vi "数字量输出自动检测_fast.vi"(11 "测试值":enum16{"0", "1"}(ring)) -> ()   [LabVIEW 2010]
uses:
  全局量/试验配置信息.vi
panel:
  in  "CAN端口":u16
  out "结束？":bool
  in  "同步_2":i32
  in  "同步_1":i32
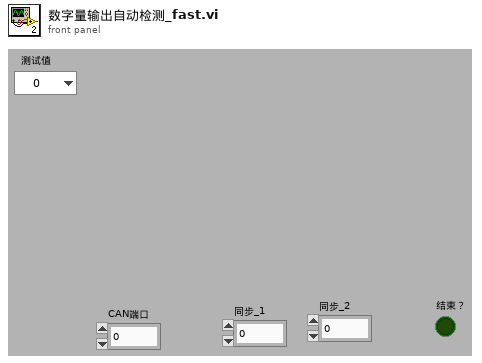
[diagram p1: front panel]
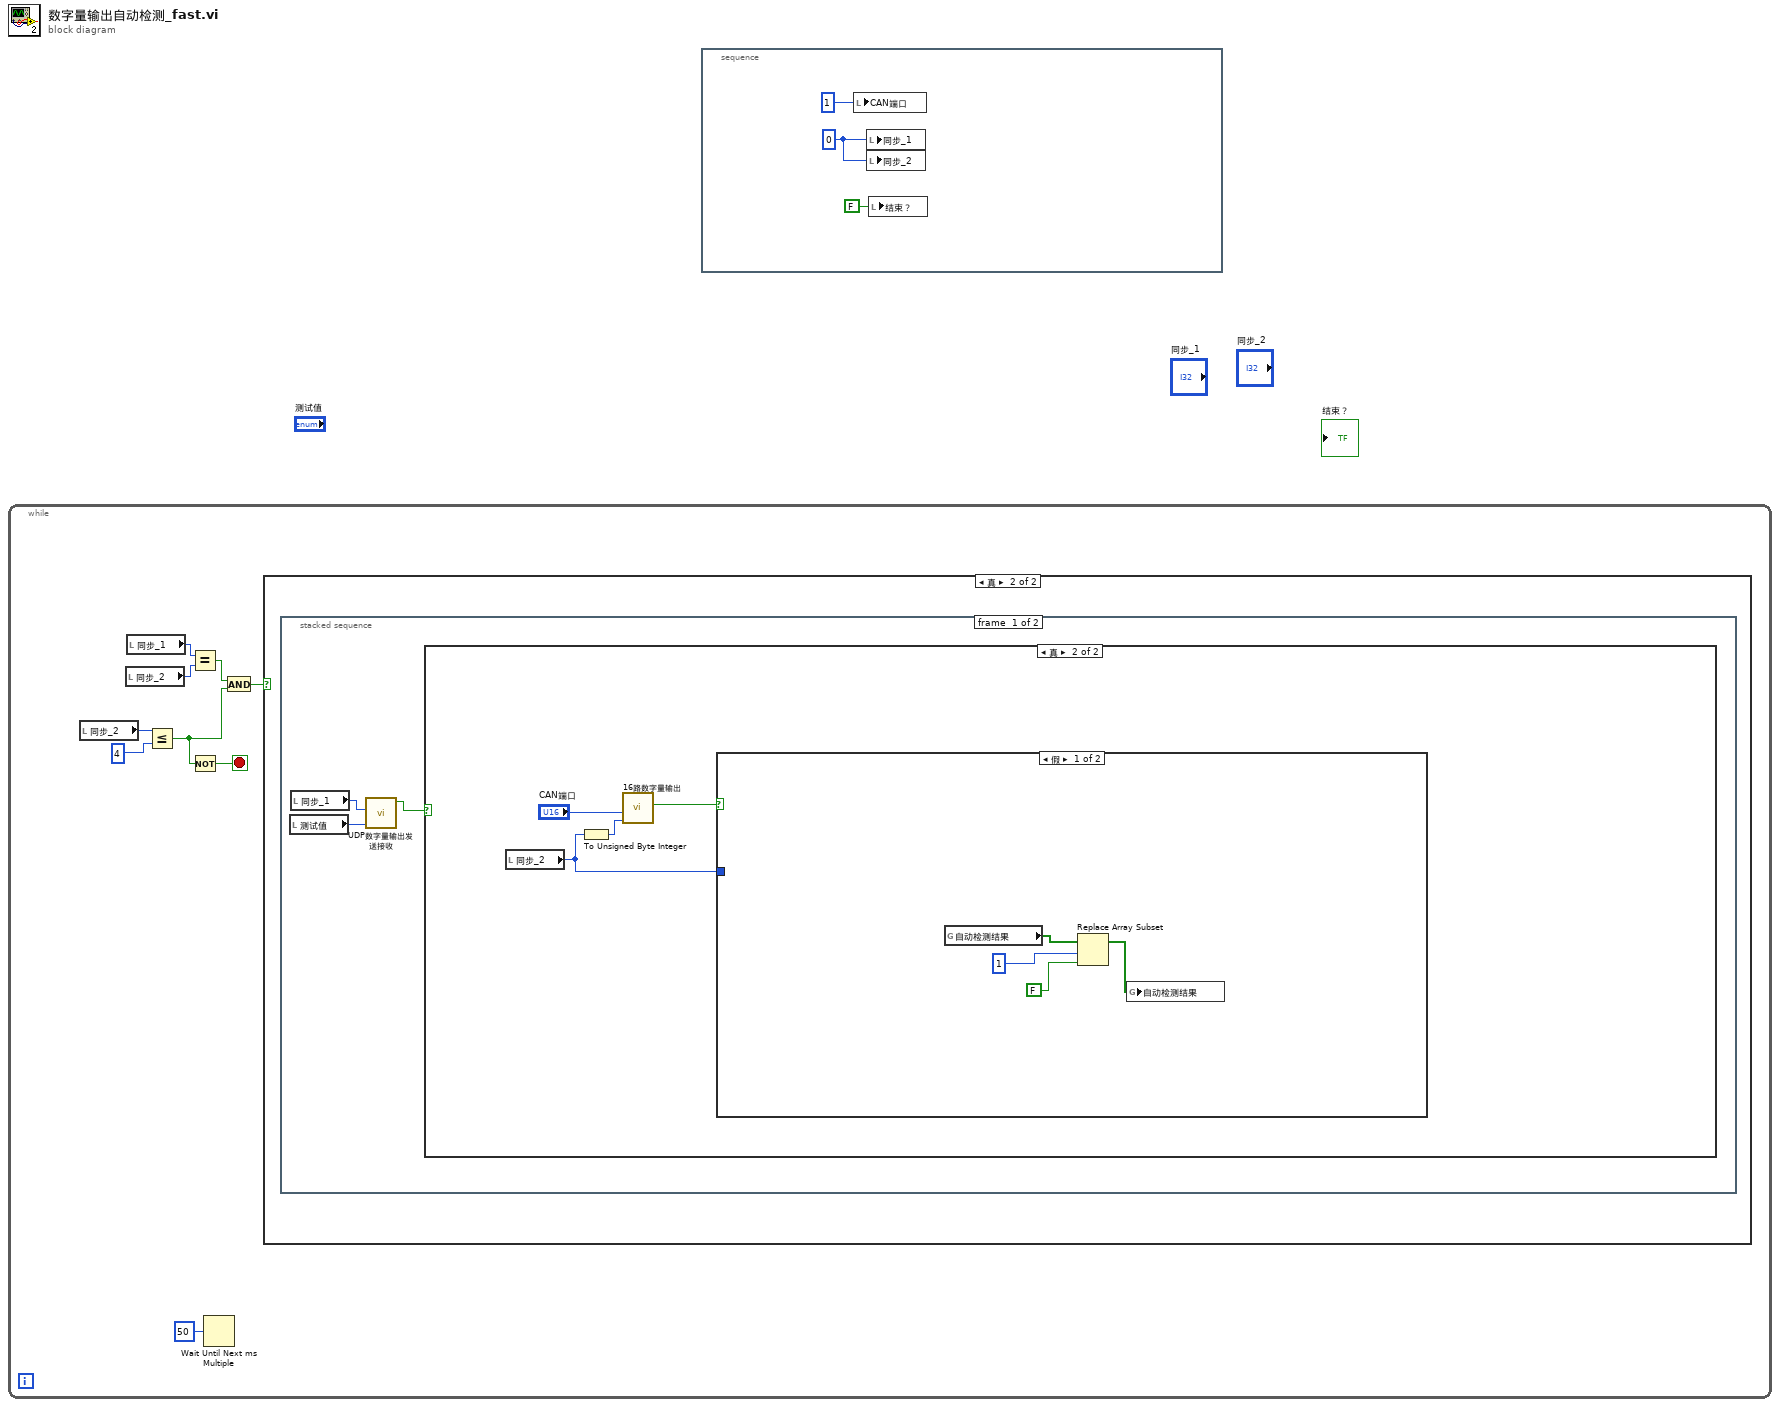
[diagram p0: block diagram]
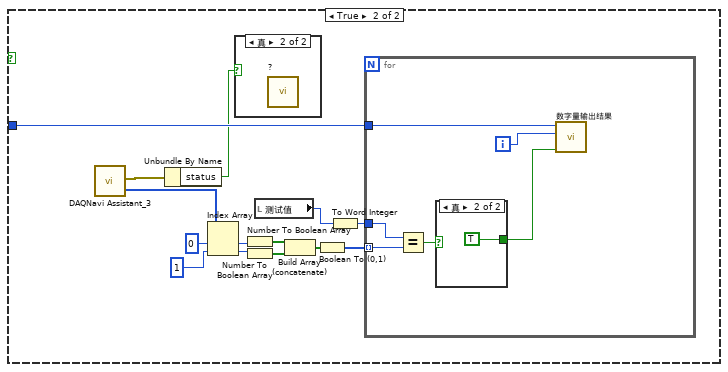
[diagram p4: hidden frame]
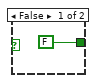
[diagram p6: hidden frame]
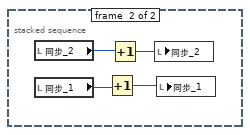
[diagram p7: hidden frame]
diagram:
  n1 = while {
    stop <- w4 stop-if-true
    n2 = local read "同步_2"() -> (w2:i32)
    n3 = local read "同步_2"() -> (w7:i32)
    n4 = local read "同步_1"() -> (w8:i32)
    n5 = Less Or Equal?(x=w2, y=4) -> (x <= y?=w3:bool)
    n6 = Equal?(x=w8, y=w7) -> (x = y?=w5:bool)
    n7 = Not(x=w3) -> (.not. x?=w4:bool)
    n8 = Wait Until Next ms Multiple(millisecond multiple=u32 50 ("毫秒倍数")) -> ()  [unwired: 1 out]
    n9 = And(x=w5, y=w3) -> (x .and. y?=w6:bool)
    n10 = case shown="真" w6 {
      frame False {
      }
      frame True {
        n11 = stacked-sequence {
          frame #0 {
            n12 = local read "测试值"() -> (w11:enum16{"0", "1"})
            n13 = local read "同步_1"() -> (w12:i32)
            n14 = call "UDP数字量输出发送接收.vi"("发送值"=w11, "第几组"=w12) -> ("正常_找到?"=w10:bool)  [unwired: 6 in, 3 out]
            n15 = case shown="真" w10 {
              frame False {
              }
              frame True {
                n16 = local read "同步_2"() -> (w16:i32)
                n17 = To Unsigned Byte Integer(number=w16) -> (unsigned 8bit integer=w14:u8)
                n18 = call "16路数字量输出.vi"("第几组数据"=w14, "CAN端口"="CAN端口") -> ("成功?"=w13:bool)  [unwired: 9 in]
                n19 = case shown="假" w13 {
                  tunnel: w16 -> [_ w34]
                  frame False {
                    n20 = global read "试验配置信息.vi" "自动检测结果"() -> (w20:bool[])
                    n21 = Replace Array Subset(array=w20, new element=FALSE, index=1 ("索引")) -> (w19:bool[])
                    n22 = global write "试验配置信息.vi" "自动检测结果"(w19) -> ()
                  }
                  frame True {
                    n23 = call "DAQNavi Assistant_3"() -> ("error out"=w26:errorcluster, "dataOut(U8Array)"=w27:u8[])  [unwired: 2 in, 16 out]
                    n24 = Unbundle By Name(w26) -> ("status"=w25:bool)
                    n25 = Index Array(array=w27, index #1=0 ("索引"), index #2=1 ("索引")) -> (element #1=w21:u8, element #2=w24:u8)
                    n26 = case shown="真" w25 {
                      frame False {
                      }
                      frame True {
                        n27 = call "?"() -> ()  [unwired: 10 in, 2 out]
                      }
                    }
                    n28 = Number To Boolean Array(number=w21) -> (Boolean array=w32:bool[])
                    n29 = Number To Boolean Array(number=w24) -> (Boolean array=w33:bool[])
                    n30 = local read "测试值"() -> (w28:enum16{"0", "1"})
                    n31 = Build Array (concatenate)(w32, w33) -> (w31:bool[])
                    n32 = Boolean To (0,1)(Boolean=w31) -> (0, 1=w30:i16[])
                    n33 = To Word Integer(number=w28) -> (16bit integer=w29:i16)
                    n34 = for {
                      tunnel: w30 -> [w38] mode=indexing
                      tunnel: w29 -> [w39]
                      tunnel: w34 -> [w37]
                      i -> [w36]
                      n35 = Equal?(x=w39, y=w38) -> (x = y?=w40:bool)
                      n36 = case shown="真" w40 {
                        tunnel: [FALSE TRUE] -> w35
                        frame False {
                        }
                        frame True {
                        }
                      }
                      n37 = call "数字量输出结果.vi"("合格?"=w35, "第几个"=w36, "第几组"=w37) -> ()  [unwired: 9 in]
                    }
                  }
                }
              }
            }
          }
          frame #1 {
            n38 = local read "同步_2"() -> (w46:i32)
            n39 = local read "同步_1"() -> (w44:i32)
            n40 = Increment(x=w44) -> (x+1=w43:i32)
            n41 = Increment(x=w46) -> (x+1=w45:i32)
            n42 = local write "同步_2"(w45) -> ()
            n43 = local write "同步_1"(w43) -> ()
          }
        }
      }
    }
  }
  n44 = stacked-sequence {
    frame #0 {
      w49 = 0 ("同步_1")
      n45 = local write "CAN端口"(u16 1 ("CAN端口")) -> ()
      n46 = local write "同步_1"(w49) -> ()
      n47 = local write "同步_2"(w49) -> ()
      n48 = local write "结束？"(FALSE ("结束？")) -> ()
    }
  }
